vi "PT Diagnostics.vi"() -> ()   [LabVIEW 2014]
uses:
  Begin/Global RefNums.vi
  <vilib>/Rock Robotics/WPI/Ultrasonic/WPI_SonarMB1010AnalogRefNum Registry Get.vi
  <vilib>/Rock Robotics/WPI/Ultrasonic/WPI_SonarMB1010AnalogGetRange.vi
panel:
  out "Switch Pressed Left":bool
  out "Switch Pressed Right":bool
  out "Sonar Left":dbl
  out "Voltage":dbl
  out "Sonar Left Side":dbl
  out "Sonar Right":dbl
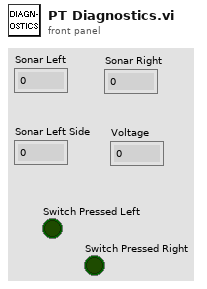
[diagram p1: front panel]
types:
  T1 = typedef "WPI_SonarMB1010AnalogDeviceRef.ctl" = cluster{"AIDeviceRef":T2, "Scaling factor (V/in)":dbl, "Average Bits":u8}
  T2 = typedef "WPI_AnalogChannelDevRef.ctl" = cluster{"DevStatus":errorcluster, "Controller":T3, "Analog Channel":T4}
  T3 = typedef "FPGA_TypedefAnalogModule.ctl" = enum16{"Controller 1"}
  T4 = typedef "FPGA_AIChannel.ctl" = enum8{"AI 0", "AI 1", "AI 2", "AI 3", "AI MXP 0", "AI MXP 1", "AI MXP 2", "AI MXP 3", "Invalid"}
  T5 = typedef "WPI_SwitchDevRef.ctl" = cluster{"DevStatus":errorcluster, "DIO Channel":T6, "Controller":T7, "CntIndex":T8, "Normally Closed":bool}
  T6 = typedef "FPGA_DIOChannel.ctl" = enum8{"DIO 0", "DIO 1", "DIO 2", "DIO 3", "DIO 4", "DIO 5", "DIO 6", "DIO 7", "DIO 8", "DIO 9", "DIO MXP 0", "DIO MXP 1", "DIO MXP 2", "DIO MXP 3", "DIO MXP 4", "DIO MXP 5", "DIO MXP 6", "DIO MXP 7", "DIO MXP 8", "DIO MXP 9", "DIO MXP 10", "DIO MXP 11", "DIO MXP 12", "DIO MXP 13", "DIO MXP 14", "DIO MXP 15", "Invalid"}
  T7 = typedef "FPGA_TypedefDigitalModule.ctl" = enum16{"Controller 1"}
  T8 = typedef "FPGA_CounterCtrSystemIndex.ctl" = enum8{"Ctr 0", "Ctr 1", "Ctr 2", "Ctr 3", "Ctr 4", "Ctr 5", "Ctr 6", "Ctr 7", "Invalid"}
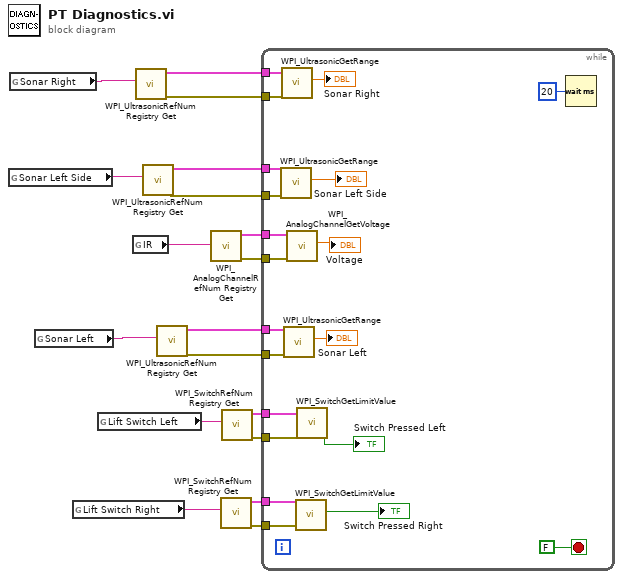
[diagram p0: block diagram]
diagram:
  n1 = global read "Global RefNums.vi" "Sonar Left Side"() -> (w6:string)
  n2 = global read "Global RefNums.vi" "Sonar Right"() -> (w3:string)
  n3 = global read "Global RefNums.vi" "Sonar Left"() -> (w10:string)
  n4 = global read "Global RefNums.vi" "Lift Switch Right"() -> (w17:string)
  n5 = global read "Global RefNums.vi" "Lift Switch Left"() -> (w18:string)
  n6 = global read "Global RefNums.vi" "IR"() -> (w7:string)
  n7 = call-poly <vilib>:"WPI_UltrasonicRefNum Registry Get.vi"("refnum name"=w3) -> ("error out"=w1:errorcluster, "SonarMB1010AnalogDevRef"=w2:T1)  [unwired: 9 in]
  n8 = call-poly <vilib>:"WPI_UltrasonicRefNum Registry Get.vi"("refnum name"=w6) -> ("error out"=w4:errorcluster, "SonarMB1010AnalogDevRef"=w5:T1)  [unwired: 9 in]
  n9 = call-poly <vilib>:"WPI_UltrasonicRefNum Registry Get.vi"("refnum name"=w10) -> ("error out"=w11:errorcluster, "SonarMB1010AnalogDevRef"=w12:T1)  [unwired: 9 in]
  n10 = call <vilib>:"WPI_AnalogChannelRefNum Registry Get.vi"("refnum name"=w7) -> ("error out"=w8:errorcluster, "AIDeviceRef"=w9:T2)  [unwired: 9 in]
  n11 = call <vilib>:"WPI_SwitchRefNum Registry Get.vi"("refnum name"=w17) -> ("error out"=w13:errorcluster, "SwitchDevRef"=w14:T5)  [unwired: 9 in]
  n12 = call <vilib>:"WPI_SwitchRefNum Registry Get.vi"("refnum name"=w18) -> ("error out"=w15:errorcluster, "SwitchDevRef"=w16:T5)  [unwired: 9 in]
  n13 = while {
    tunnel: w16 -> [w37]
    tunnel: w15 -> [w36]
    tunnel: w14 -> [w35]
    tunnel: w13 -> [w34]
    tunnel: w12 -> [w30]
    tunnel: w11 -> [w29]
    tunnel: w9 -> [w27]
    tunnel: w8 -> [w26]
    tunnel: w5 -> [w24]
    tunnel: w4 -> [w23]
    tunnel: w2 -> [w21]
    tunnel: w1 -> [w20]
    stop <- FALSE stop-if-true
    n14 = call-poly <vilib>:"WPI_UltrasonicGetRange.vi"("error in"=w23, "SonarMB1010AnalogDevRef"=w24) -> ("Distance"=→"Sonar Left Side":dbl)  [unwired: 7 in, 2 out]
    n15 = call-poly <vilib>:"WPI_UltrasonicGetRange.vi"("error in"=w20, "SonarMB1010AnalogDevRef"=w21) -> ("Distance"=→"Sonar Right":dbl)  [unwired: 7 in, 2 out]
    n16 = call-poly <vilib>:"WPI_UltrasonicGetRange.vi"("error in"=w29, "SonarMB1010AnalogDevRef"=w30) -> ("Distance"=→"Sonar Left":dbl)  [unwired: 7 in, 2 out]
    n17 = call <vilib>:"WPI_AnalogChannelGetVoltage.vi"("error in (no error)"=w26, "AIDeviceRef"=w27) -> ("Voltage"=→"Voltage":dbl)  [unwired: 7 in, 2 out]
    n18 = call <vilib>:"WPI_SwitchGetLimitValue.vi"("error in (no error)"=w34, "SwitchDevRef"=w35) -> ("Switch Pressed"=→"Switch Pressed Right":bool)  [unwired: 7 in, 2 out]
    n19 = call <vilib>:"WPI_SwitchGetLimitValue.vi"("error in (no error)"=w36, "SwitchDevRef"=w37) -> ("Switch Pressed"=→"Switch Pressed Left":bool)  [unwired: 7 in, 2 out]
    n20 = Wait (ms)(milliseconds to wait=u32 20) -> ()  [unwired: 1 out]
  }
